vi "CRYAPI Win Move.vi"(6 "Mouse LButton In":bool, 8 "ToolBar Click In":bool, 9 "StartPositin In":T1, 10 "MousePositin In":T1, 11 "VI Ref In":refnum<vi>) -> (0 "ToolBar Click Out":bool, 1 "StartPositin Out":T1, 3 "VI Ref Out":refnum<vi>)   [LabVIEW 2013]
uses:
  <vilib>/Utility/miscctls.llb/LVRectTypeDef.ctl
panel:
  out "Start_Positin 2":T1
  in  "ToolBar Click":bool
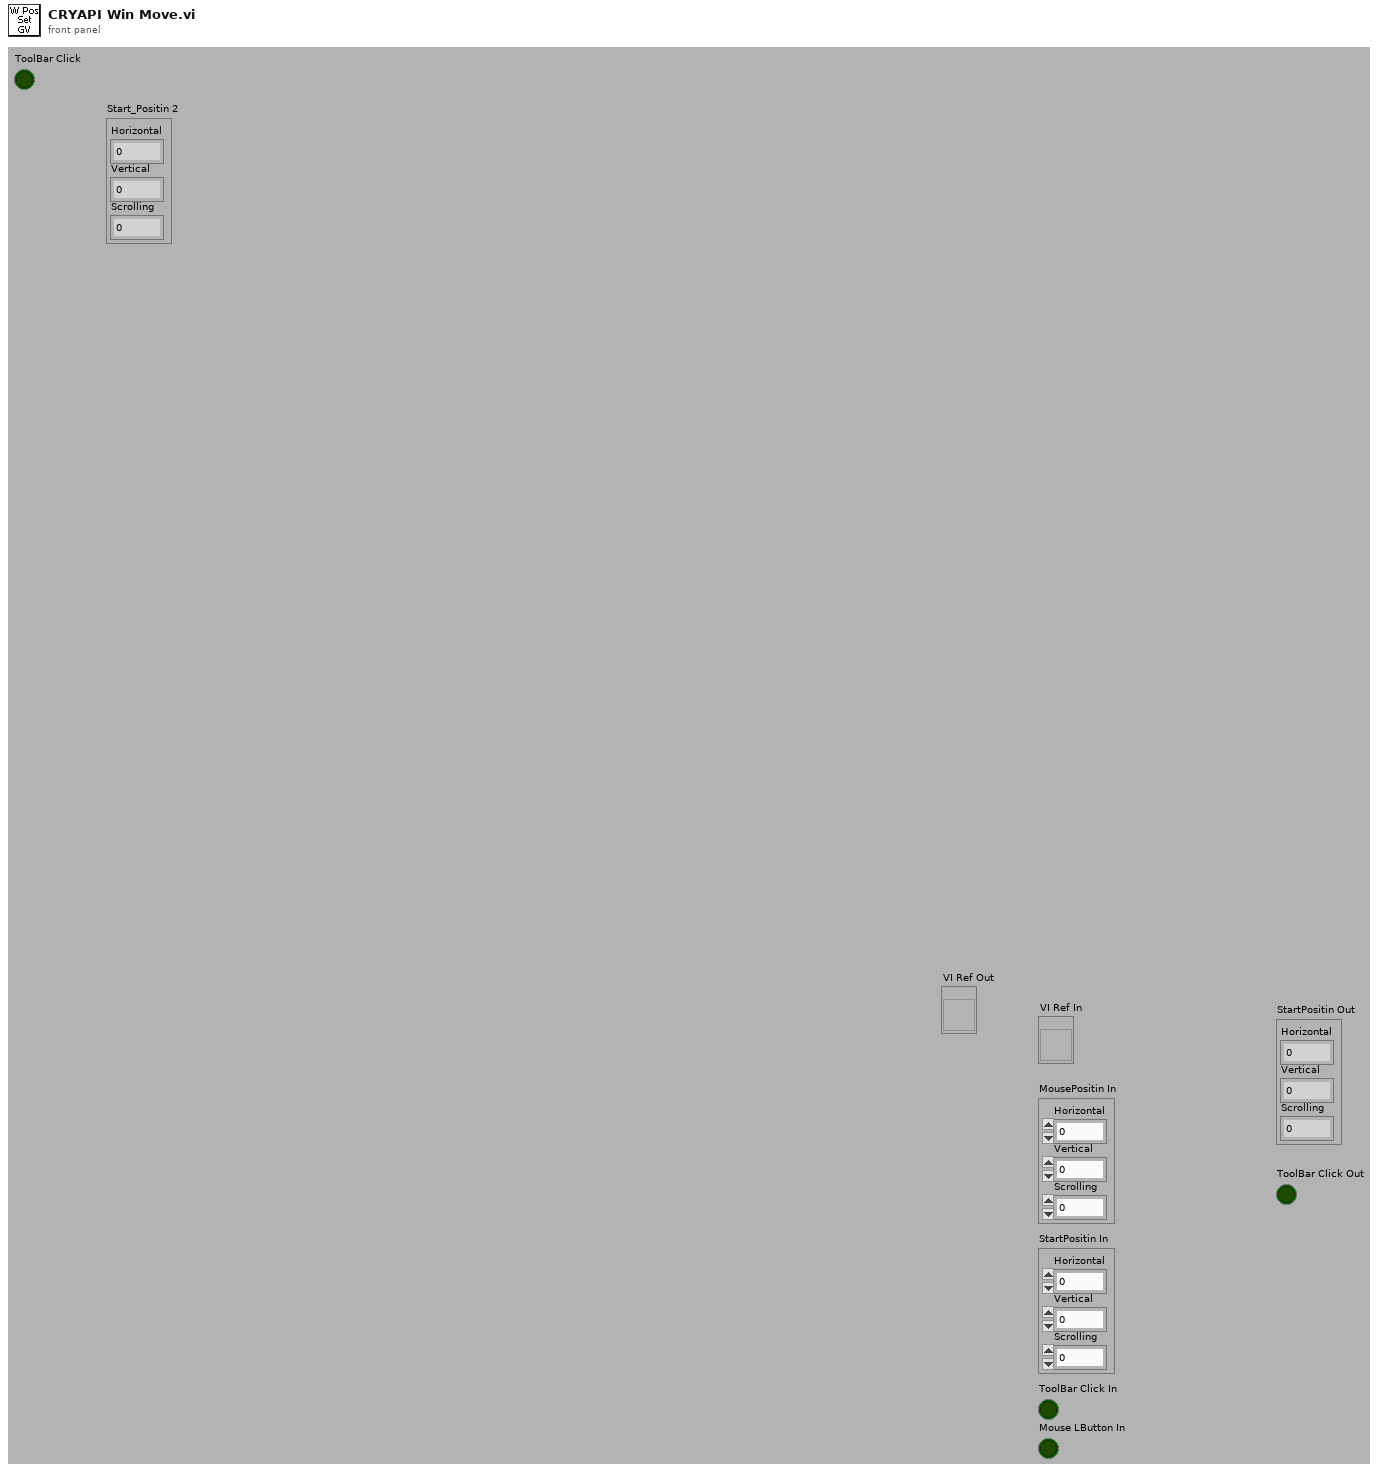
[diagram p1: front panel]
types:
  T1 = cluster{"Horizontal":i32, "Vertical":i32, "Scrolling":i32}
  T2 = typedef "LVRectTypeDef.ctl" = cluster{"Left":i16, "Top":i16, "Right":i16, "Bottom":i16}
  T3 = cluster{"Left":i16, "Top":i16, "Width":i16, "Height":i16}
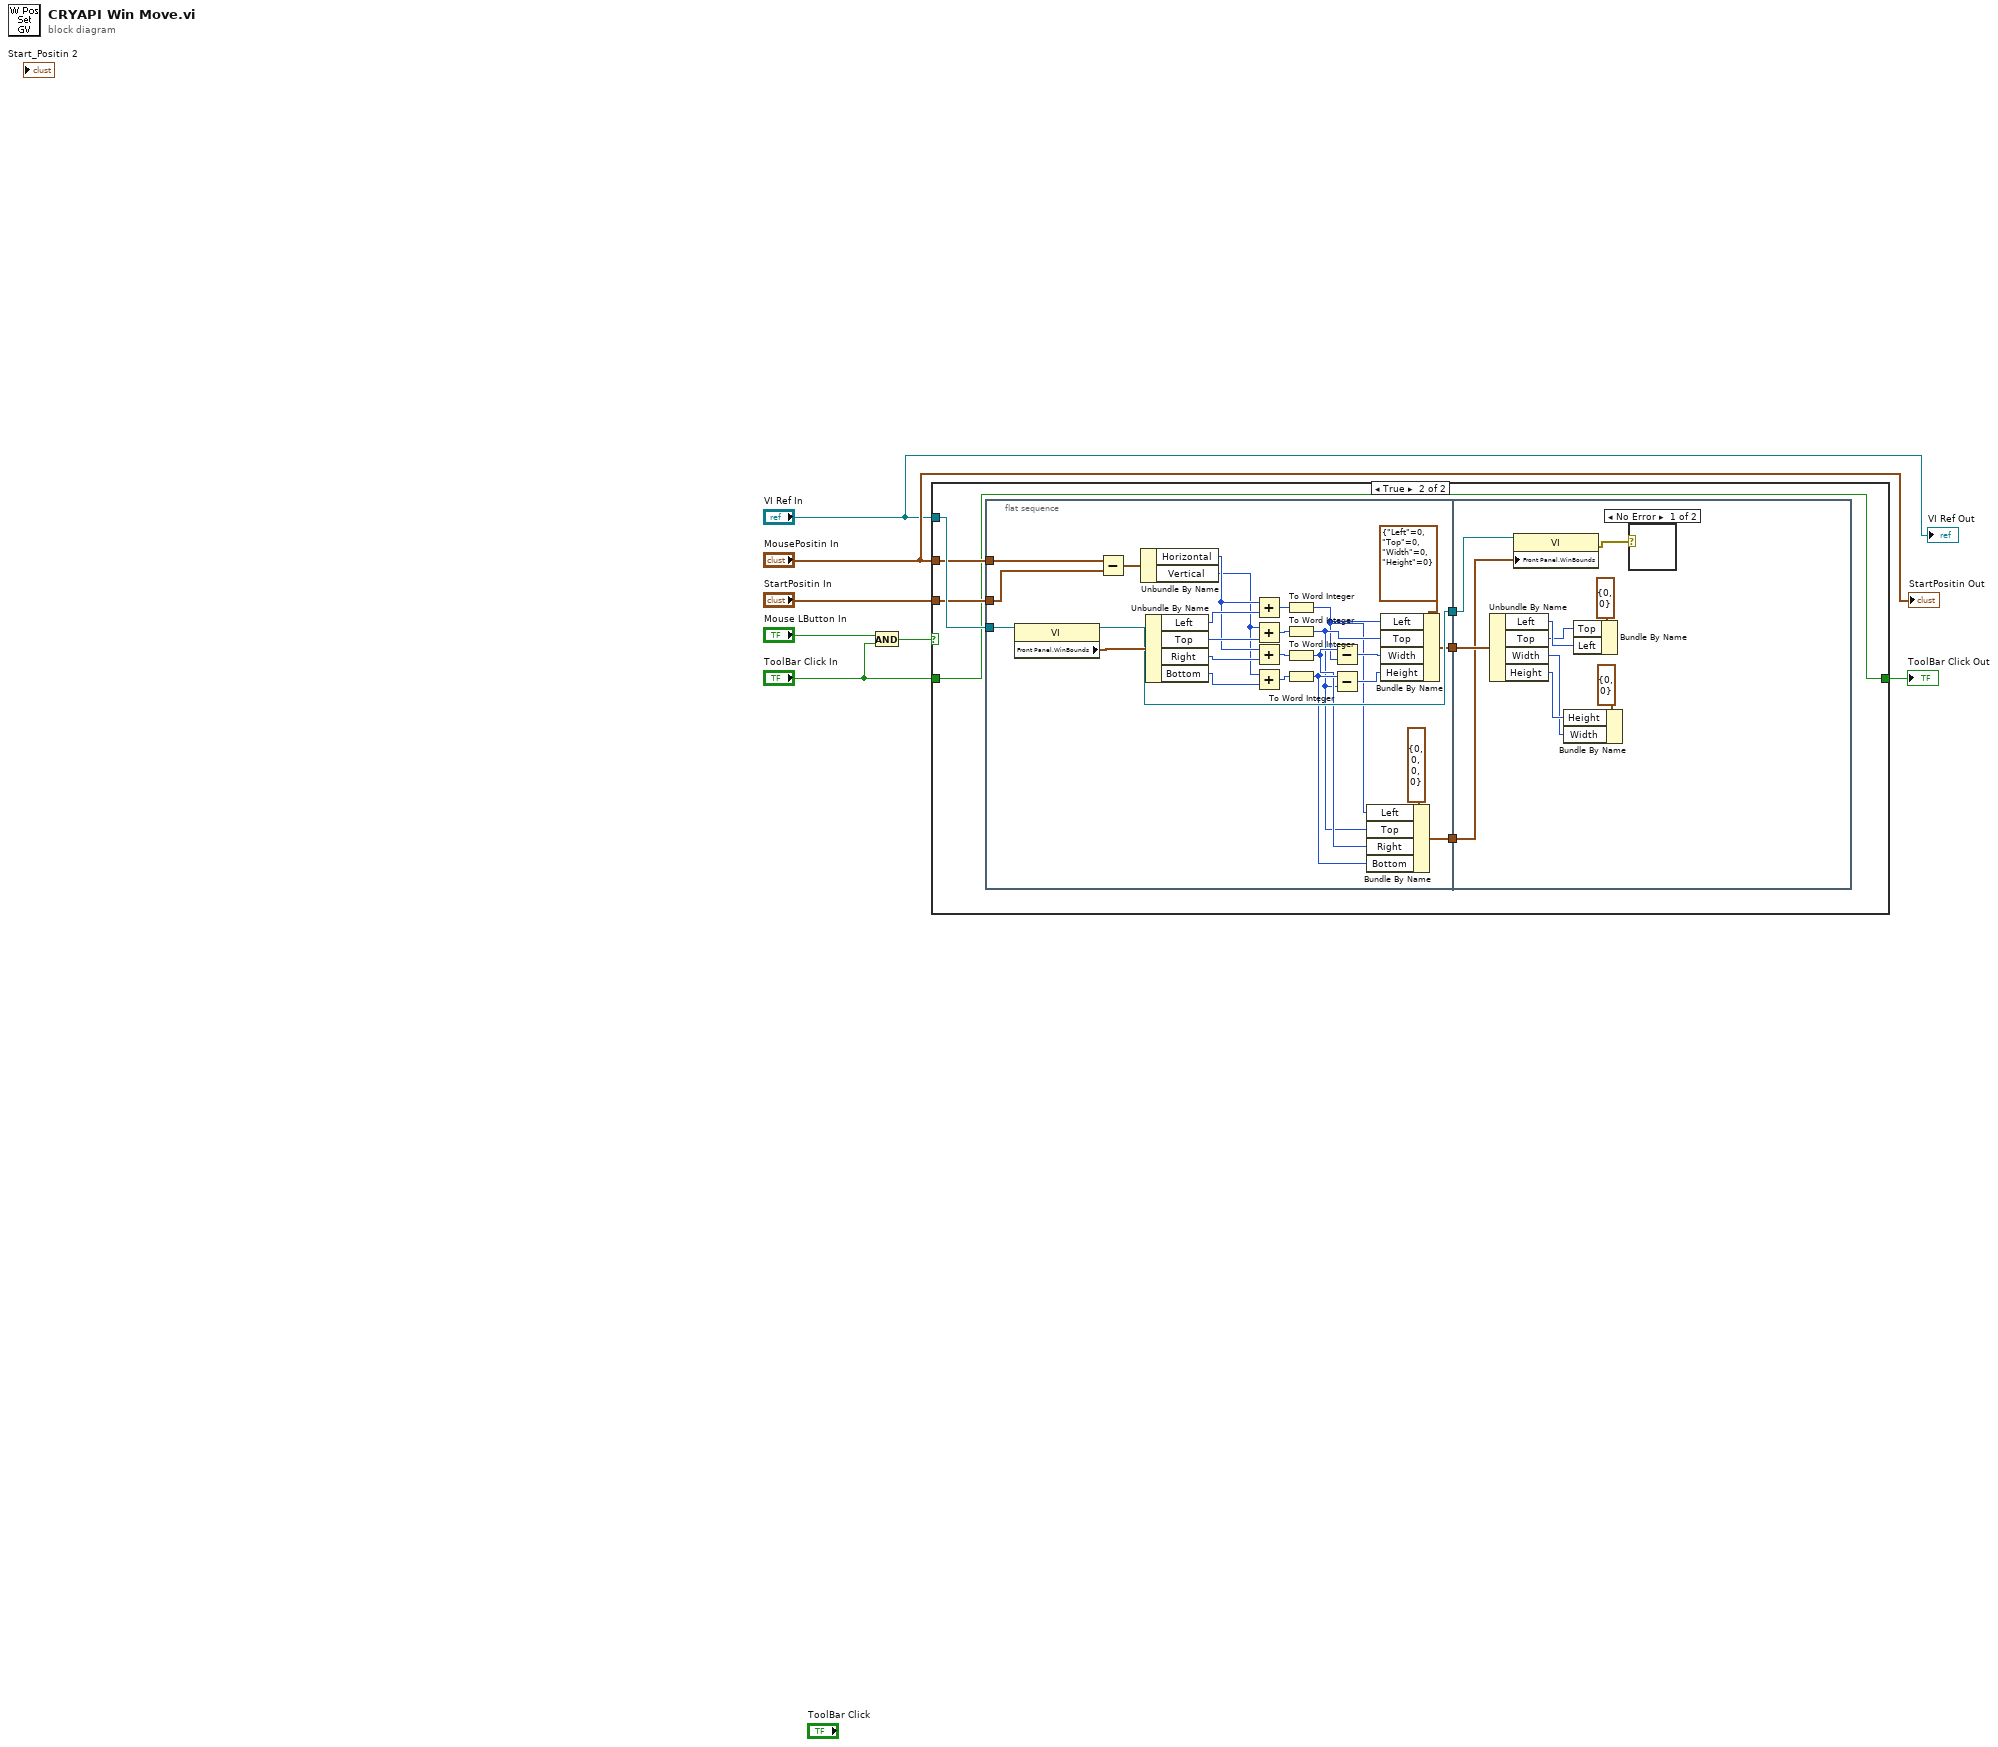
[diagram p0: block diagram]
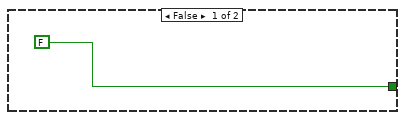
[diagram p2: hidden frame]
diagram:
  n1 = And(x="Mouse LButton In", y="ToolBar Click In") -> (x .and. y?=w7:bool)
  n2 = case shown="True" w7 {
    tunnel: "VI Ref In" -> [_ w13]
    tunnel: "MousePositin In" -> [_ w12]
    tunnel: [FALSE ("TitlebarMouse Down") w10] -> w5
    tunnel: "StartPositin In" -> [_ w11]
    tunnel: "ToolBar Click In" -> [_ w10]
    frame False {
    }
    frame True {
      n3 = flat-sequence {
        tunnel: w12 -> [w29]
        tunnel: [w24] -> w15
        tunnel: [w30] -> w14
        tunnel: w13 -> [w28]
        tunnel: w11 -> [w27]
        tunnel: [w16] -> w9
        tunnel: w15 -> [w51]
        tunnel: w14 -> [w48]
        tunnel: w9 -> [w43]
        frame #0 {
          n4 = property class="VI"(reference=w28) -> (reference out=w30:refnum<vi>, "Front Panel.WinBounds"=w41:T2)  [unwired: 1 in, 1 out]
          n5 = Subtract(x=w29, y=w27) -> (x-y=w26:T1)
          n6 = Unbundle By Name(w26) -> ("Horizontal"=w36:i32, "Vertical"=w35:i32)
          n7 = Unbundle By Name(w41) -> ("Left"=w40:i16, "Top"=w39:i16, "Right"=w38:i16, "Bottom"=w37:i16)
          n8 = Add(x=w36, y=w40) -> (x+y=w34:i32)
          n9 = Add(x=w35, y=w39) -> (x+y=w33:i32)
          n10 = Add(x=w36, y=w38) -> (x+y=w32:i32)
          n11 = Add(x=w35, y=w37) -> (x+y=w31:i32)
          n12 = To Word Integer(number=w34) -> (16bit integer=w17:i16)
          n13 = To Word Integer(number=w33) -> (16bit integer=w18:i16)
          n14 = To Word Integer(number=w32) -> (16bit integer=w19:i16)
          n15 = To Word Integer(number=w31) -> (16bit integer=w20:i16)
          n16 = Subtract(x=w19, y=w17) -> (x-y=w23:i16)
          n17 = Subtract(x=w20, y=w18) -> (x-y=w22:i16)
          n18 = Bundle By Name(cluster=T2 {"Left"=0, "Top"=0, "Right"=0, "Bottom"=0} ("Front Panel Window:Window Bounds"), "Left"=w17, "Top"=w18, "Right"=w19, "Bottom"=w20) -> (w16:T2)
          n19 = Bundle By Name(cluster=T3 {"Left"=0, "Top"=0, "Width"=0, "Height"=0}, "Left"=w17, "Top"=w18, "Width"=w23, "Height"=w22) -> (w24:T3)
        }
        frame #1 {
          n20 = Unbundle By Name(w51) -> ("Left"=w45:i16, "Top"=w44:i16, "Width"=w46:i16, "Height"=w47:i16)
          n21 = property class="VI"(reference=w48, "Front Panel.WinBounds"=w43) -> (error out=w42:errorcluster)  [unwired: 1 in, 1 out]
          n22 = Bundle By Name(cluster=cluster{"Height":i16, "Width":i16} {"Height"=0, "Width"=0} ("Size"), "Height"=w47, "Width"=w46) -> ()  [unwired: 1 out]
          n23 = Bundle By Name(cluster=cluster{"Top":i16, "Left":i16} {"Top"=0, "Left"=0} ("Position"), "Top"=w44, "Left"=w45) -> ()  [unwired: 1 out]
          n24 = case shown="No Error" w42 {
            frame No Error {
            }
            frame Error {
            }
          }
        }
      }
    }
  }
  "ToolBar Click Out" <- w5
  "StartPositin Out" <- "MousePositin In"
  "VI Ref Out" <- "VI Ref In"
